vi "DllFxpSinhAndCosh.vi"(6 "ready for output":bool, 8 "input valid":bool, 11 "Phase":fxp<+,1,1>) -> (0 "output valid":bool, 2 "Cosh":fxp<+,1,1>, 3 "Sinh":fxp<+,1,1>, 4 "ready for input":bool)   [LabVIEW 2017]
uses:
  <vilib>/rvi/FXPMathLib/FxpSinhAndCosh/subVIs/nifxpmath_SinhAndCosh_SimConfig.ctl
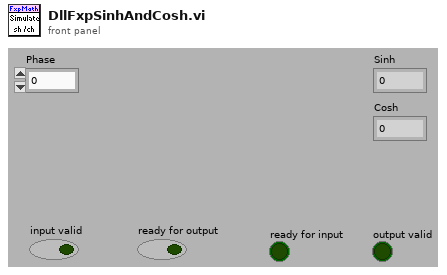
[diagram p1: front panel]
types:
  T1 = typedef "nifxpmath_SinhAndCosh_SimConfig.ctl" = cluster{"kPhaseLen":u16, "kPhaseIwl":i16, "kPhaseSigned":bool, "kSinhCoshLen":u16, "InputRegister":bool, "OutputRegister":bool, "kPrecision":u16, "kIteration":u16, "QuantiMode":u16, "HandShake":bool, "CycleLimit":u16, "StrictLimit":bool}
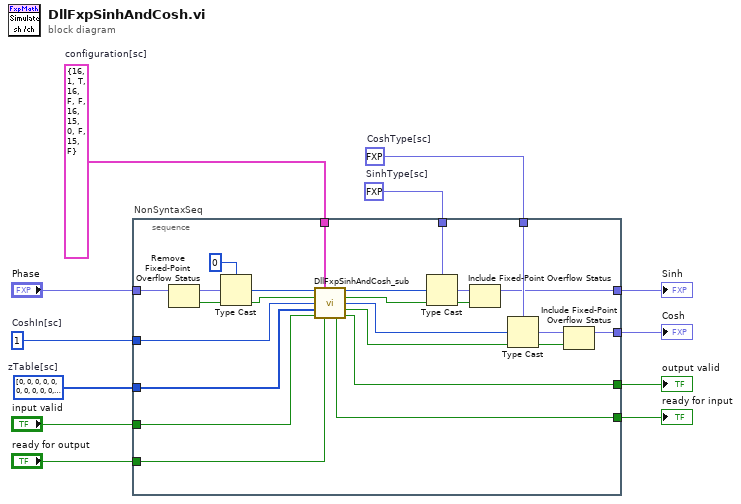
[diagram p0: block diagram]
diagram:
  w1 = T1 {"kPhaseLen"=16, "kPhaseIwl"=1, "kPhaseSigned"=TRUE, "kSinhCoshLen"=16, "InputRegister"=FALSE, "OutputRegister"=FALSE, "kPrecision"=16, "kIteration"=15, "QuantiMode"=0, "HandShake"=FALSE, "CycleLimit"=15, "StrictLimit"=FALSE}  # configuration[sc]
  w6 = fxp<+,1,1> 0.0  # CoshType[sc]
  w7 = fxp<+,1,1> 0.0  # SinhType[sc]
  w9 = u64[] [0, 0, 0, 0, 0, 0, 0, 0, 0, 0, 0, 0, 0, 0, 0, 0]  # zTable[sc]
  w10 = u64 1  # CoshIn[sc]
  n1 = stacked-sequence "NonSyntaxSeq" {
    tunnel: "Phase" -> [w28]
    tunnel: "input valid" -> [w24]
    tunnel: w10 -> [w26]
    tunnel: w9 -> [w25]
    tunnel: [w19] -> w8
    tunnel: w7 -> [w33]
    tunnel: w6 -> [w32]
    tunnel: [w16] -> w5
    tunnel: w1 -> [w31]
    tunnel: "ready for output" -> [w23]
    tunnel: [w14] -> w3
    tunnel: [w13] -> w2
    frame #0 {
      n2 = Remove Fixed-Point Overflow Status(3:w28) -> (0:w27:bool, 1:w29:fxp<+,1,1>)
      n3 = Type Cast(type=u64 0, x=w29) -> (*(type *) &x=w30:u64)
      n4 = call <vilib>:"DllFxpSinhAndCosh_sub.vi"("phase"=w30, "configuration[sc]"=w31, "phase ovfl status"=w27, "CoshIn"=w26, "ztable"=w25, "input valid"=w24, "ready for output"=w23) -> ("sinh"=w22:u64, "sinh ovfl status"=w20:bool, "cosh"=w18:u64, "cosh ovfl status"=w15:bool, "ready for input"=w13:bool, "output valid"=w14:bool)  [unwired: 3 out]
      n5 = Type Cast(type=w33, x=w22) -> (*(type *) &x=w21:fxp<+,1,1>)
      n6 = Include Fixed-Point Overflow Status(2:w20, 3:w21) -> (1:w19:fxp<+,1,1>)
      n7 = Type Cast(type=w32, x=w18) -> (*(type *) &x=w17:fxp<+,1,1>)
      n8 = Include Fixed-Point Overflow Status(2:w15, 3:w17) -> (1:w16:fxp<+,1,1>)
    }
  }
  "output valid" <- w3
  "ready for input" <- w2
  "Sinh" <- w8
  "Cosh" <- w5
